vi "cc_io.vi"(3 "error in (no error)":errorcluster, 4 "Output Command":string, 5 "VISA In":refnum<visa-resource-name>) -> (0 "error out":errorcluster, 1 "Input String":string, 2 "VISA out":refnum<visa-resource-name>)   [LabVIEW 2020]
doc: "Cryocon Output then Input VI.\nWrites a command string to an open instrument, then reads the response.\nThe ERROR VI is called to handle any input/output errors."
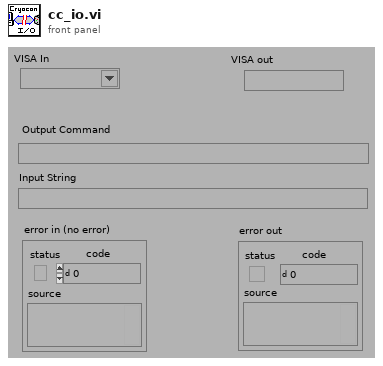
[diagram p1: front panel]
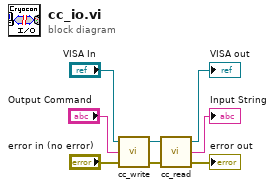
[diagram p0: block diagram]
diagram:
  n1 = call "cc_write.vi"("error in (no error)"="error in (no error)", "Output Command"="Output Command", "VISA In"="VISA In") -> ("error out"=w7:errorcluster, "VISA Out"=w8:refnum<visa-resource-name>)  [unwired: 1 in]
  n2 = call "cc_read.vi"("error in (no error)"=w7, "VISA In"=w8) -> ("error out"=→"error out":errorcluster, "Input String"=→"Input String":string, "VISA Out"=→"VISA out":refnum<visa-resource-name>)  [unwired: 1 in]
